vi "Close XWPF Reader.vi"(8 "error in (no error)":errorcluster, 11 "xwpfReader in":refnum<class "xwpfReader.lvclass">) -> (0 "error out":errorcluster, 3 "xwpfReader out":refnum<class "xwpfReader.lvclass">)   [LabVIEW 2017, in "LabVIEW NPOI.lvlib" / "xwpfReader.lvclass"]
doc: "Closes XWPFDocuement and FlieStream references."
uses:
  xwpfReader.lvclass
  xwpfReader.lvclass/xwpfReader.ctl
  Support/File Stream/File Stream.lvlib
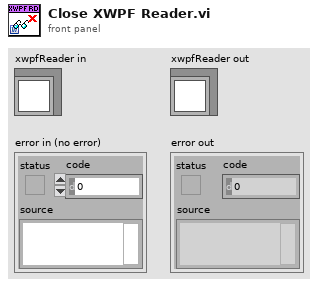
[diagram p1: front panel]
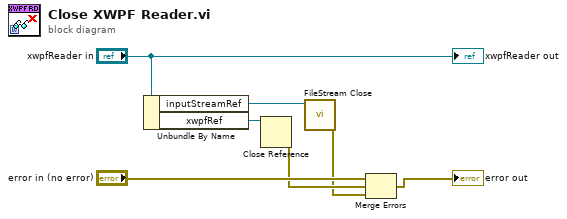
[diagram p0: block diagram]
diagram:
  n1 = Unbundle By Name("xwpfReader in") -> ("inputStreamRef"=w2:refnum<k24>, "xwpfRef"=w5:refnum<k24>)
  n2 = Close Reference(reference=w5) -> (error out=w3:errorcluster)  [unwired: 1 in]
  n3 = call "FileStream Close.vi"("reference"=w2) -> ("error out"=w1:errorcluster)  [unwired: 10 in]
  n4 = Merge Errors("error in (no error)", w3, w1) -> (→"error out":errorcluster)
  "xwpfReader out" <- "xwpfReader in"
